vi "testMemoryDefault.vi"(8 "error in (no error)":errorcluster, 11 "TestCase in":refnum<class "Memory Manager Unit Tests.lvclass">) -> (0 "error out":errorcluster, 3 "TestCase out":refnum<class "Memory Manager Unit Tests.lvclass">)   [LabVIEW 2016, in "Memory Manager Unit Tests.lvclass"]
uses:
  Memory Manager Unit Tests.lvclass
  Library/Classes/Pointer.Internal/Memory.Pointer.Internal.lvclass
  C:/Git/Personal/LabVIEW-Memory-Manager/Source/Library/Classes/Pointer/Memory.Pointer.lvclass
  Library/Classes/Pointer/Memory.Pointer.lvclass/Memory.Pointer.ctl
  Library/Classes/Pointer/Accessors/Get Address.vi
  Library/Classes/Pointer/Accessors/Get Size.vi
  <vilib>/addons/_JKI Toolkits/VI Tester/TestCase.llb/TestCase.lvclass
  C:/Program Files (x86)/National Instruments/LabVIEW 2016/vi.lib/addons/_JKI Toolkits/VI Tester/TestCase.llb/TestCase.lvclass
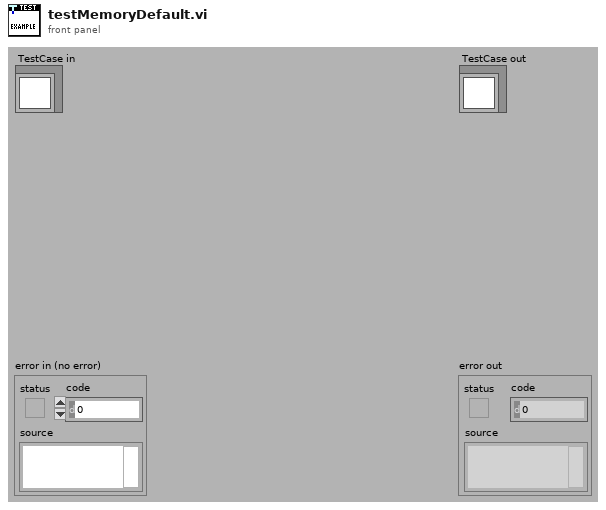
[diagram p1: front panel]
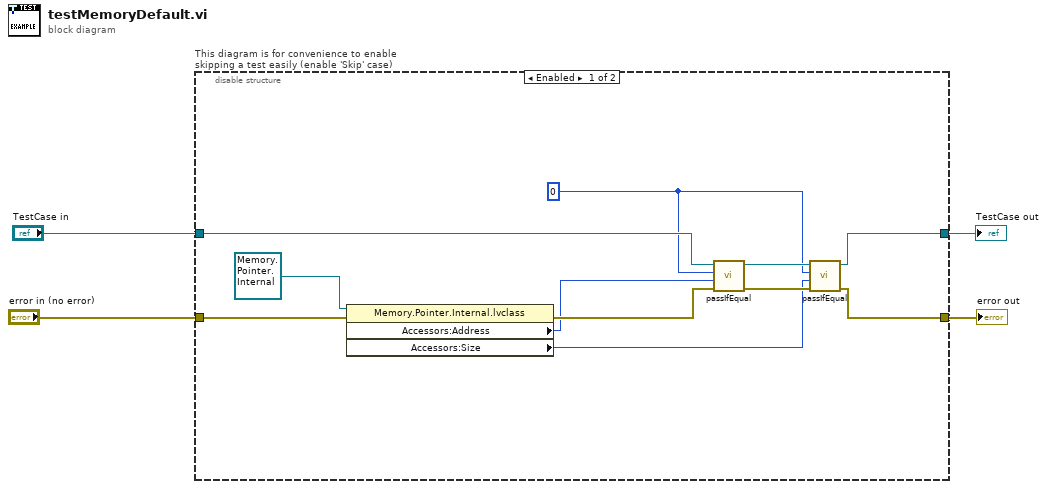
[diagram p0: block diagram]
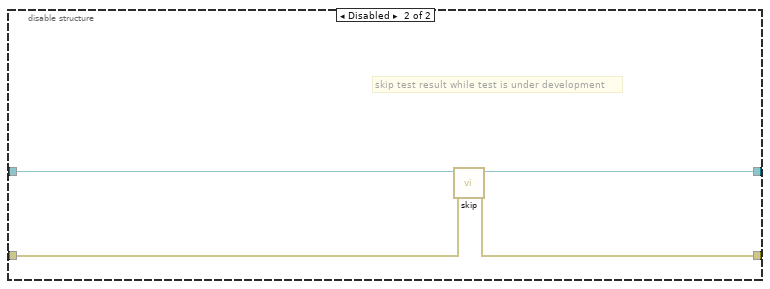
[diagram p2: hidden frame]
diagram:
  n1 = disable-structure "This diagram is for convenience to enable skipping a test easily (enable 'Skip' case)" shown="Enabled" {
    disable-tunnel: "TestCase in" -> [w15 w19]
    disable-tunnel: [w9 w17] -> w1
    disable-tunnel: [w7 w18] -> w3
    disable-tunnel: "error in (no error)" -> [w14 w16]
    frame Enabled {
      w6 = u64 0 ("Address")
      n2 = property class="Memory.Pointer.Internal.lvclass"(reference=refnum<class "Memory.Pointer.Internal.lvclass"> refnum ("pointer"), error in=w14) -> (error out=w13:errorcluster, "Accessors:Address"=w11:u64, "Accessors:Size"=w5:u64)  [unwired: 1 out]
      n3 = call-dynamic "passIfEqual.vi"("error in (no error)"=w13, "y"=w11, "x"=w6, "TestCase in"=w15) -> ("error out"=w8:errorcluster, "TestCase out"=w10:refnum<class "Memory Manager Unit Tests.lvclass">)  [unwired: 6 in]
      n4 = call-dynamic "passIfEqual.vi"("error in (no error)"=w8, "y"=w5, "x"=w6, "TestCase in"=w10) -> ("error out"=w7:errorcluster, "TestCase out"=w9:refnum<class "Memory Manager Unit Tests.lvclass">)  [unwired: 6 in]
    }
    frame Disabled {
      # "skip test result while test is under development"
      n5 = call <vilib>:"skip.vi"("error in (no error)"=w16, "TestCase in"=w19) -> ("error out"=w18:errorcluster, "TestCase out"=w17:refnum<class "Memory Manager Unit Tests.lvclass">)  [unwired: 8 in]
    }
  }
  "error out" <- w3
  "TestCase out" <- w1
